vi "Configure Resistor Interface.vi"(8 "error in (no error)":errorcluster, 9 "Number of Bands in":u8=4 min=3 max=6 step=1, 10 "Enum Refnum":refnum<vi>[](array[refnum]), 11 "Color Box Refnum":refnum<vi>[](array[refnum])) -> (0 "error out":errorcluster)   [LabVIEW 2018, in "Front Panel Interface.lvlib"]
uses:
  Front Panel Interface.lvlib
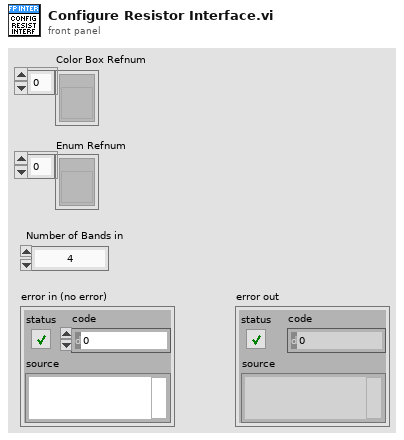
[diagram p1: front panel]
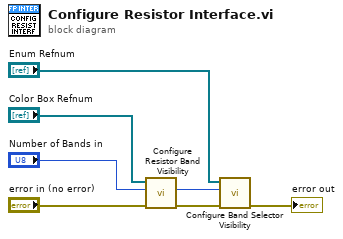
[diagram p0: block diagram]
diagram:
  n1 = call "Configure Resistor Band Visibility.vi"("error in (no error)"="error in (no error)", "Number of Bands in"="Number of Bands in", "Color Box Refnum"="Color Box Refnum") -> ("error out"=w7:errorcluster, "Number of Bands out"=w6:u8)  [unwired: 7 in]
  n2 = call "Configure Band Selector Visibility.vi"("error in (no error)"=w7, "Number of Bands in"=w6, "Enum Refnum"="Enum Refnum") -> ("error out"=→"error out":errorcluster)  [unwired: 7 in, 1 out]
